vi "Path_HDH Dependency Finder Target Folder.vi"() -> (2 "Success?":bool, 3 "HDH\\VIPM path":path)   [LabVIEW 2019, in "Project.Dependencies Finder.lvlib"]
uses:
  Project.Dependencies Finder.lvlib
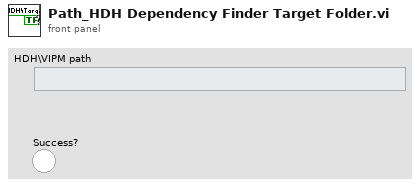
[diagram p1: front panel]
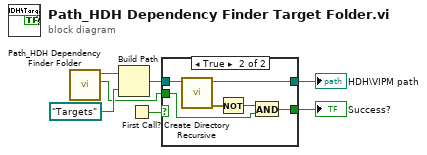
[diagram p0: block diagram]
diagram:
  n1 = call "Path_HDH Dependency Finder Folder.vi"() -> ("Success?"=w1:bool, "HDH\\VIPM path"=w6:path)  [unwired: 10 in]
  n2 = Build Path(base path=w6, name or relative path=path "Targets") -> (appended path=w4:path)
  n3 = First Call?() -> (First Call?: T/F=w7:bool)
  n4 = case shown="True" w7 {
    tunnel: w4 -> [w9 w14]
    tunnel: [w9 w13] -> w3
    tunnel: [w8 w10] -> w2
    tunnel: w1 -> [w8 w12]
    frame False {
    }
    frame True {
      n5 = call <vilib>:"Create Directory Recursive.vi"("directory"=w14) -> ("error out"=w15:errorcluster, "directory copy"=w13:path)  [unwired: 4 in, 1 out]
      n6 = Not(x=w15) -> (.not. x?=w11:bool)
      n7 = And(x=w11, y=w12) -> (x .and. y?=w10:bool)
    }
  }
  "HDH\\VIPM path" <- w3
  "Success?" <- w2
